vi "Prompt User for File Path to Load From.vi"(8 "error in (no error)":errorcluster, 11 "Message Enqueuer in":refnum<class "Message Enqueuer.lvclass">) -> (0 "error out":errorcluster, 3 "Message Enqueuer out":refnum<class "Message Enqueuer.lvclass">)   [LabVIEW 2017, in "Measurement UI.lvlib" / "Prompt User for File Path to Load From.lvclass"]
uses:
  Prompt User for File Path to Load From.lvclass
  <vilib>/ActorFramework/Message Enqueuer/Message Enqueuer.lvclass
  C:/Program Files (x86)/National Instruments/LabVIEW 2017/vi.lib/ActorFramework/Message/Message.lvclass
  <vilib>/ActorFramework/Message Enqueuer/Message Enqueuer.lvclass/Message Enqueuer.ctl
  <vilib>/ActorFramework/Message Priority Queue/Priority Enqueue.vi
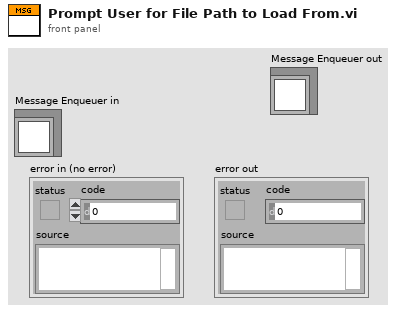
[diagram p1: front panel]
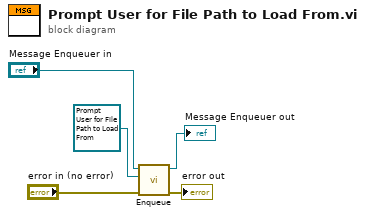
[diagram p0: block diagram]
diagram:
  n1 = call <vilib>:"Enqueue.vi"("error in (no error)"="error in (no error)", "Message"=refnum<class "Prompt User for File Path to Load From.lvclass"> refnum ("Prompt User for File Path to Load From.lvclass"), "Message Enqueuer in"="Message Enqueuer in") -> ("error out"=→"error out":errorcluster, "Message Enqueuer out"=→"Message Enqueuer out":refnum<class "Message Enqueuer.lvclass">)  [unwired: 7 in]
